vi "ARMS_2.vi"() -> ()   [LabVIEW 2018]
uses:
  <vilib>/Analysis/Matrix/Datatypes/RealMatrix.ctl
  <vilib>/Analysis/Matrix/NI_Matrix.lvlib
panel:
  in  "Phi":dbl(slide) scale=0.0..5.0
  out "Array":dbl[](array[numeric])
  in  "stop":bool
  out "A x B 2":T1=[[1.0, 0.0, 0.0, 0.0], [0.0, 6.123233995736766e-17, 1.0, 0.0], [0.0, -1.0, 6.123233995736766e-17, 0.0], [0.0, 0.0, 0.0, 1.0]] format="%#_2g"
  out "3D Picture 3":refnum<vi>(3d-picture)
  in  "X":dbl(slide) scale=0.0..2.0
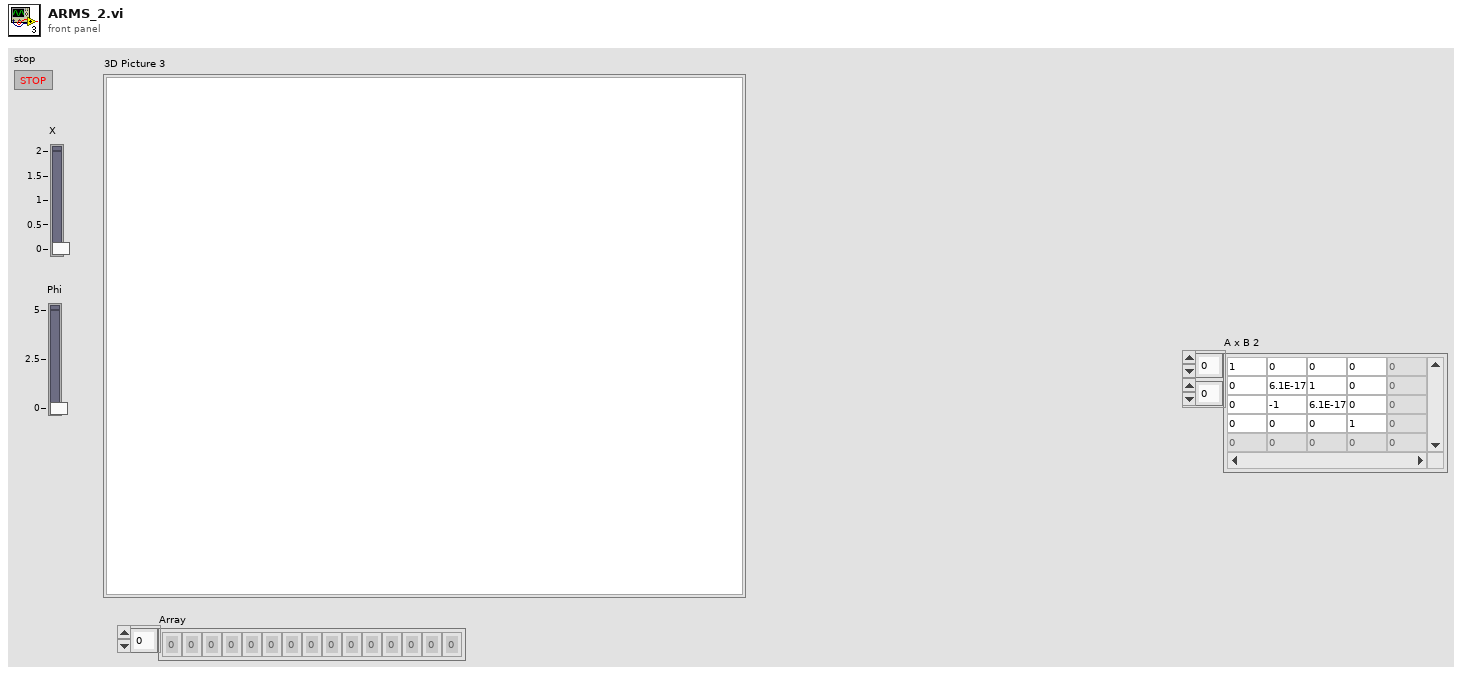
[diagram p1: front panel]
types:
  T1 = typedef "NI_Matrix.lvlib/RealMatrix.ctl" = dbl[][]
  T2 = cluster{"Theta":dbl, "d":dbl, "a":dbl, "alpha (degrees)":dbl}[]
  T3 = cluster{"Theta":dbl, "d":dbl, "a":dbl, "alpha (degrees)":dbl}
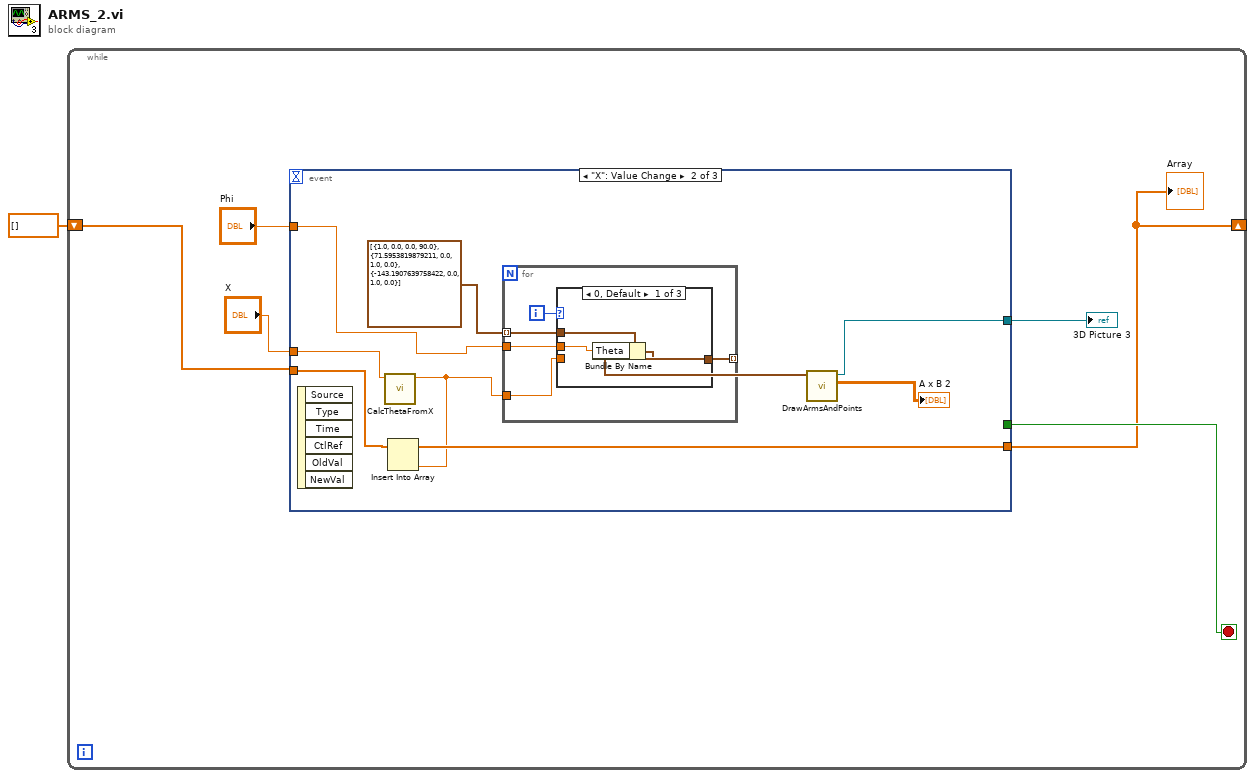
[diagram p0: block diagram]
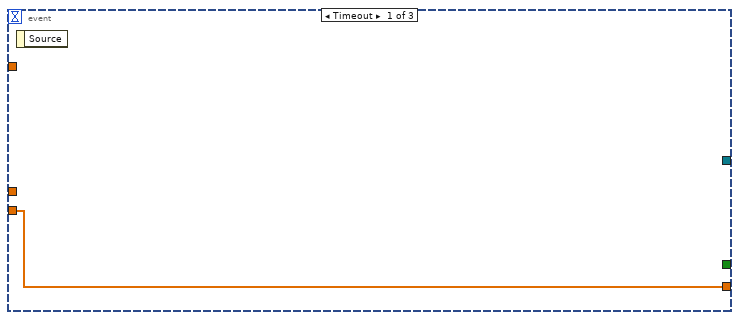
[diagram p2: hidden frame]
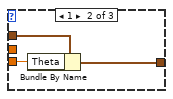
[diagram p3: hidden frame]
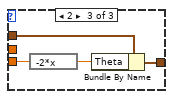
[diagram p4: hidden frame]
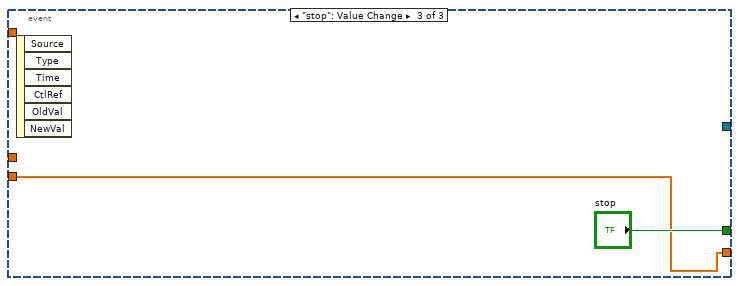
[diagram p5: hidden frame]
diagram:
  n1 = while {
    shift-right: [w3] -> _
    shift-left: dbl[] [] -> [w4]
    stop <- w5 stop-if-true
    n2 = event shown="[1] \"X\": Value Change" {
      selector: _ -> [_ _ _]
      dyn-events: _ -> [_ _ _]
      timeout: _ -> [_ _ _]
      tunnel: "X" -> [_ w17 _]
      tunnel: [_ w14 _] -> w6
      tunnel: [_ _ "stop"] -> w5
      tunnel: [w8 w11 w33] -> w3
      tunnel: w4 -> [w8 w12 w33]
      tunnel: "Phi" -> [_ w9 _]
      event Timeout {
        n3 = event-data() -> ()  [unwired: 1 in, 1 out]
      }
      event "X": Value Change {
        n4 = event-data() -> ()  [unwired: 1 in, 6 out]
        n5 = call "CalcThetaFromX.vi"("X"=w17) -> ("Numeric"=w10:dbl)  [unwired: 10 in]
        n6 = Insert Into Array(array=w12, new element=w10) -> (w11:dbl[])  [unwired: 1 in]
        n7 = for {
          tunnel: w10 -> [w21]
          tunnel: T2 [{"Theta"=1.0, "d"=0.0, "a"=0.0, "alpha (degrees)"=90.0}, {"Theta"=71.5953819879211, "d"=0.0, "a"=1.0, "alpha (degrees)"=0.0}, {"Theta"=-143.1907639758422, "d"=0.0, "a"=1.0, "alpha (degrees)"=0.0}] ("Joints") -> [w20] mode=indexing
          tunnel: [w19] -> w15 mode=indexing
          tunnel: w9 -> [w18]
          i -> [w22]
          n8 = case shown="0, Default" w22 {
            tunnel: w21 -> [_ w27 w31]
            tunnel: w20 -> [w25 w28 w32]
            tunnel: [w23 w26 w30] -> w19
            tunnel: w18 -> [w24 _ _]
            frame 0, Default {
              n9 = Bundle By Name(cluster=w25, "Theta"=w24) -> (w23:T3)
            }
            frame 1 {
              n10 = Bundle By Name(cluster=w28, "Theta"=w27) -> (w26:T3)
            }
            frame 2 {
              n11 = expression code="-2*x"(w31) -> (w29:dbl)
              n12 = Bundle By Name(cluster=w32, "Theta"=w29) -> (w30:T3)
            }
          }
        }
        n13 = call "DrawArmsAndPoints.vi"("Array"=w15) -> ("A x B"=→"A x B 2":T1, "SceneObject out"=w14:refnum<vi>)  [unwired: 9 in]
      }
      event "stop": Value Change {
        n14 = event-data() -> ()  [unwired: 1 in, 6 out]
      }
    }
    "3D Picture 3" <- w6
    "Array" <- w3
  }
